vi "RF Data to Bytes.vi"(1 "Y":cdb[](array[numeric]), 2 "attributes":variant) -> (0 "Bytes":i32)   [LabVIEW 2021]
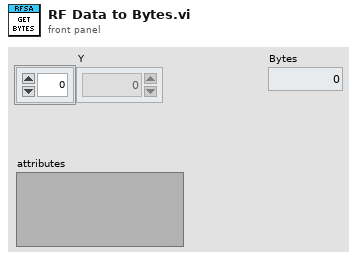
[diagram p1: front panel]
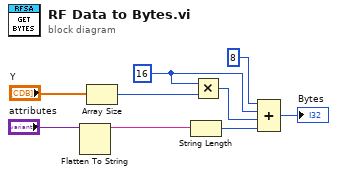
[diagram p0: block diagram]
diagram:
  w8 = 16 ("x")
  n1 = Flatten To String(anything="attributes") -> (data string=w3:string)  [unwired: 3 in, 2 out]
  n2 = Array Size(array="Y") -> (size(s)=w1:i32)
  n3 = String Length(string=w3) -> (length=w5:i32)
  n4 = Multiply(x=w8, y=w1) -> (x*y=w6:i32)
  n5 = Compound Arithmetic op=ADD(8 ("value"), w8, w6, w5) -> (→"Bytes":i32)
